vi "Chebyshev Approximation.vi"(4 "number of points":u32=5, 5 "formula":string, 6 "order":u32=3, 7 "end":dbl=1.0 format="%.2f", 8 "start":dbl format="%.2f") -> (0 "error":i32, 1 "Y":dbl[](array[numeric]) format="%.2f", 2 "X":dbl[](array[numeric]) format="%.2f", 3 "C":dbl[](array[numeric]) format="%.2f")   [LabVIEW 2010, in "NI_Gmath.lvlib"]
doc: "Determines a given function using Chebyshev polynomials."
uses:
  NI_Gmath.lvlib
panel:
  # "Example:\n\n number of points: 100 \n start: 0.0 \n end: 1.0\n order: 5 \n formula: (x-(3/10))^2+sin(x)"
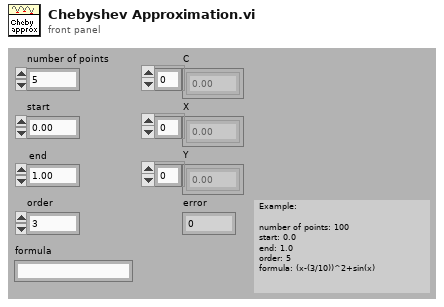
[diagram p1: front panel]
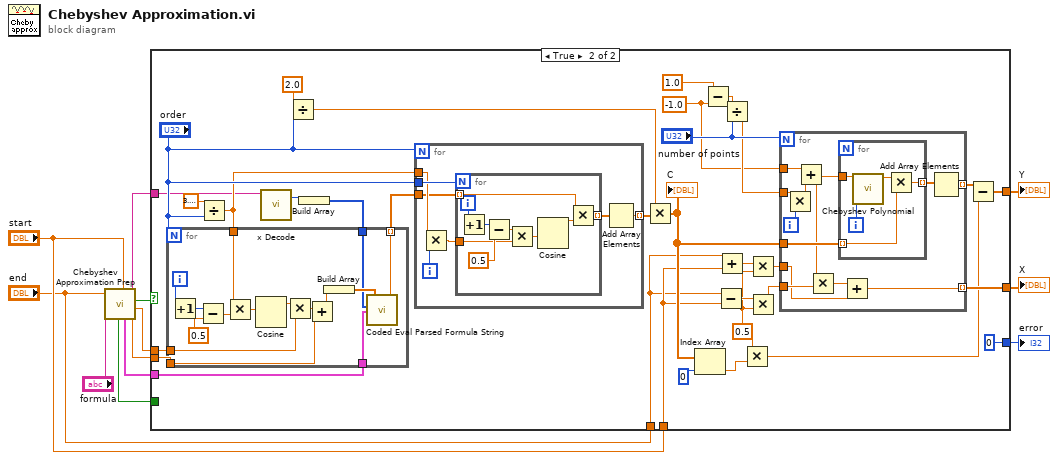
[diagram p0: block diagram]
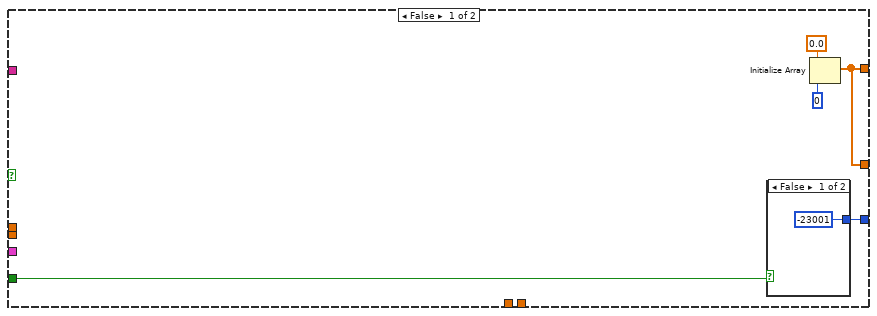
[diagram p2: hidden frame]
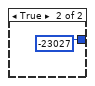
[diagram p3: hidden frame]
diagram:
  n1 = call "Chebyshev Approximation Prep.vi"("start"="start", "formula"="formula", "end"="end") -> ("value 2"=w11:dbl, "Parsed Formula"=w3:cluster{"Table":i32[][], "Y Values":dbl[]}, "value 1"=w12:dbl, "error (general)"=w6:bool, "x string"=w7:string, "error situation"=w4:bool)
  n2 = case shown="True" w6 {
    tunnel: w11 -> [_ w50]
    tunnel: w12 -> [_ w49]
    tunnel: [w15 w28] -> w10
    tunnel: [w15 w25] -> w9
    tunnel: w7 -> [_ w24]
    tunnel: [w13 0] -> w5
    tunnel: w4 -> [w14 _]
    tunnel: w3 -> [_ w22]
    tunnel: "start" -> [_ w21]
    tunnel: "end" -> [_ w20]
    frame False {
      n3 = case shown="False" w14 {
        tunnel: [-23001 -23027] -> w13
        frame False {
        }
        frame True {
        }
      }
      n4 = Initialize Array(0.0, 0) -> (w15:dbl[])
    }
    frame True {
      w44 = 0.5
      w41 = -1.0
      n5 = Divide(x=3.141592653589793, y="order") -> (x/y=w30:dbl)
      n6 = call "x Decode.vi"("x string"=w24) -> ("number"=w31:i32)  [unwired: 1 in, 1 out]
      n7 = Divide(x=2.0, y="order") -> (x/y=w35:dbl)
      n8 = Build Array(w31) -> (w32:i32[])
      n9 = for {
        N: "order" -> [_]
        tunnel: w30 -> [w98]
        tunnel: w32 -> [w87]
        tunnel: [w95] -> w48 mode=indexing
        tunnel: w49 -> [w93]
        tunnel: w50 -> [w90]
        tunnel: w22 -> [w86]
        i -> [w99]
        n10 = Increment(x=w99) -> (x+1=w94:i32)
        n11 = Subtract(x=w94, y=0.5) -> (x-y=w97:dbl)
        n12 = Multiply(x=w98, y=w97) -> (x*y=w96:dbl)
        n13 = Cosine(x=w96) -> (cos(x)=w92:dbl)
        n14 = Multiply(x=w92, y=w93) -> (x*y=w91:dbl)
        n15 = Add(x=w91, y=w90) -> (x+y=w89:dbl)
        n16 = Build Array(w89) -> (w88:dbl[])
        n17 = call "Coded Eval Parsed Formula String.vi"("Parsed Formula"=w86, "Variables"=w87, "X Values"=w88) -> ("y value"=w95:dbl)  [unwired: 1 in, 1 out]
      }
      n18 = for {
        N: "order" -> [_]
        tunnel: "order" -> [w76]
        tunnel: w30 -> [w75]
        tunnel: w48 -> [w73]
        tunnel: [w71] -> w36 mode=indexing
        i -> [w70]
        n19 = Multiply(x=w75, y=w70) -> (x*y=w74:dbl)
        n20 = for {
          N: w76 -> [_]
          tunnel: w74 -> [w77]
          tunnel: w73 -> [w84] mode=indexing
          tunnel: [w83] -> w72 mode=indexing
          i -> [w82]
          n21 = Increment(x=w82) -> (x+1=w78:i32)
          n22 = Subtract(x=w78, y=0.5) -> (x-y=w80:dbl)
          n23 = Multiply(x=w80, y=w77) -> (x*y=w79:dbl)
          n24 = Cosine(x=w79) -> (cos(x)=w85:dbl)
          n25 = Multiply(x=w84, y=w85) -> (x*y=w83:dbl)
        }
        n26 = Add Array Elements(numeric array=w72) -> (sum=w71:dbl)
      }
      n27 = Multiply(x=w35, y=w36) -> (x*y=w51:dbl[])
      "C" <- w51
      n28 = Index Array(array=w51, index=0) -> (element=w39:dbl)
      n29 = Subtract(x=1.0, y=w41) -> (x-y=w37:dbl)
      n30 = Subtract(x=w20, y=w21) -> (x-y=w45:dbl)
      n31 = Add(x=w20, y=w21) -> (x+y=w43:dbl)
      n32 = Divide(x=w37, y="number of points") -> (x/y=w42:dbl)
      n33 = Multiply(x=w44, y=w39) -> (x*y=w26:dbl)
      n34 = Multiply(x=w43, y=w44) -> (x*y=w46:dbl)
      n35 = Multiply(x=w45, y=w44) -> (x*y=w47:dbl)
      n36 = for {
        N: "number of points" -> [_]
        tunnel: w42 -> [w64]
        tunnel: w41 -> [w62]
        tunnel: w51 -> [w60]
        tunnel: [w58] -> w27 mode=indexing
        tunnel: [w53] -> w28 mode=indexing
        tunnel: w46 -> [w54]
        tunnel: w47 -> [w56]
        i -> [w63]
        n37 = Multiply(x=w64, y=w63) -> (x*y=w61:dbl)
        n38 = Add(x=w62, y=w61) -> (x+y=w57:dbl)
        n39 = Multiply(x=w57, y=w56) -> (x*y=w55:dbl)
        n40 = for {
          tunnel: w57 -> [w66]
          tunnel: w60 -> [w68] mode=indexing
          tunnel: [w67] -> w59 mode=indexing
          i -> [w65]
          n41 = call "Chebyshev Polynomial.vi"("n"=w65, "x"=w66) -> ("T(n,x)"=w69:dbl)
          n42 = Multiply(x=w69, y=w68) -> (x*y=w67:dbl)
        }
        n43 = Add(x=w55, y=w54) -> (x+y=w53:dbl)
        n44 = Add Array Elements(numeric array=w59) -> (sum=w58:dbl)
      }
      n45 = Subtract(x=w27, y=w26) -> (x-y=w25:dbl[])
    }
  }
  "X" <- w10
  "Y" <- w9
  "error" <- w5
